vi "Get All Folder VI Data.vi"(8 "error in":errorcluster, 11 "Path":path) -> (0 "error out":errorcluster, 2 "Tree Map out":refnum<class "Tree Map.lvclass">, 3 "VI Data Map":T1)   [LabVIEW 2023, in "VI Properties Editor.lvlib"]
doc: "Gets all VI data from a folder located at <B>Path</B>."
uses:
  VI Properties Editor.lvlib
  Tree Map/Tree Map/Tree Map.lvclass
  <vilib>/picture/picture.llb/imagedata.ctl
  CTLs/VI Properties.ctl
  CTLs/Control Properties.ctl
  CTLs/VI Data Map.ctl
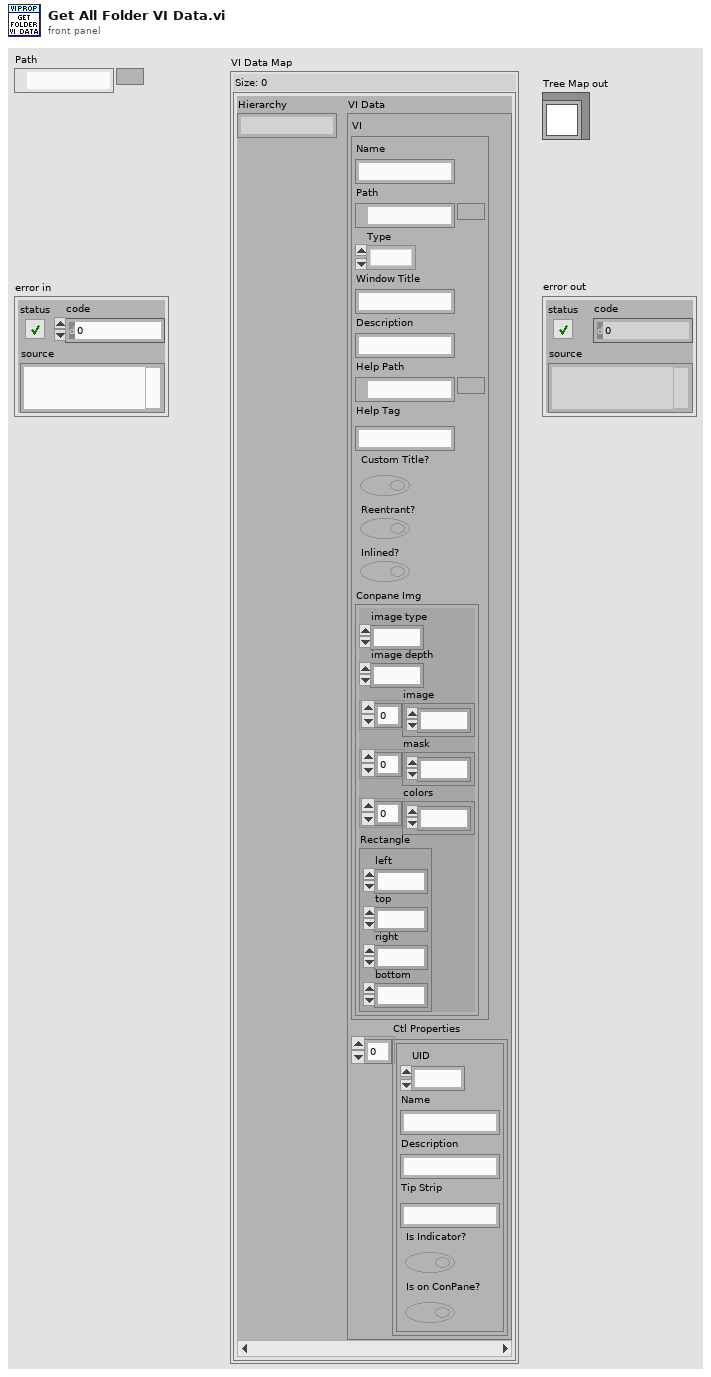
[diagram p1: front panel]
types:
  T1 = typedef "VI Properties Editor.lvlib/VI Data Map.ctl" = map{string, cluster{"VI":T2, "Ctl Properties":T4[]}}
  T2 = typedef "VI Properties Editor.lvlib/VI Properties.ctl" = cluster{"Name":string, "Path":path, "Type":enum32{"invalid VI type", "Standard VI", "Control VI", "Global VI", "Polymorphic VI", "Configuration VI", "SubSystem", "Facade VI", "Method VI", "Statechart Diagram VI"}, "Window Title":string, "Description":string, "Help Path":path, "Help Tag":string, "Custom Title?":bool, "Reentrant?":bool, "Inlined?":bool, "Conpane Img":T3}
  T3 = typedef "imagedata.ctl" = cluster{"image type":i32, "image depth":i32, "image":u8[], "mask":u8[], "colors":u32[], "Rectangle":cluster{"left":i16, "top":i16, "right":i16, "bottom":i16}}
  T4 = typedef "VI Properties Editor.lvlib/Control Properties.ctl" = cluster{"UID":i32, "Name":string, "Description":string, "Tip Strip":string, "Is Indicator?":bool, "Is on ConPane?":bool}
  T5 = typedef "VI Properties Editor.lvlib/VI Data.ctl" = cluster{"VI":T2, "Ctl Properties":T4[]}
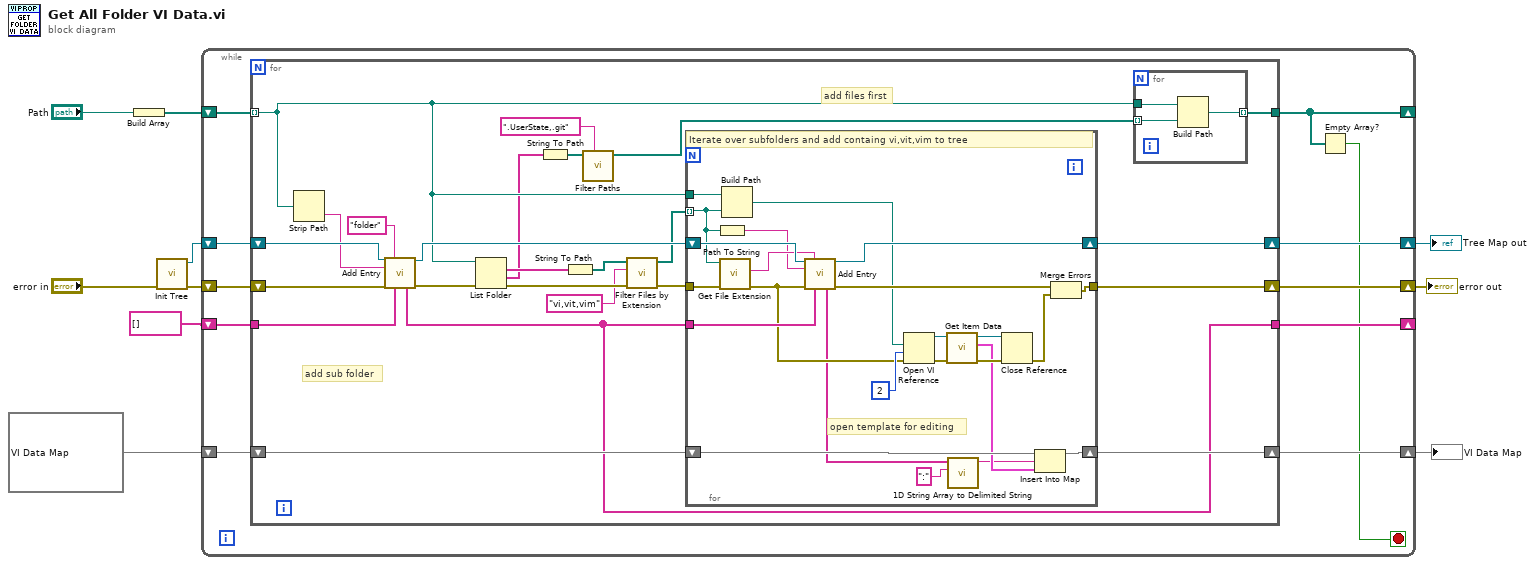
[diagram p0: block diagram]
diagram:
  n1 = Build Array("Path") -> (w3:path[])
  n2 = call "Init Tree.vi"("error in"="error in") -> ("error out"=w7:errorcluster, "Tree Map out"=w6:refnum<class "Tree Map.lvclass">)  [unwired: 9 in]
  n3 = while {
    shift-right: [w21] -> w10
    shift-left: w7 -> [w18]
    shift-right: [w20] -> w9
    shift-left: T1 {} ("VI Data Map") -> [w19]
    shift-right: [w15] -> w5
    shift-left: w6 -> [w16]
    shift-right: [w12] -> _
    shift-left: w3 -> [w14]
    shift-right: [w13] -> _
    shift-left: string[] [] ("Hierarchy") -> [w17]
    stop <- w11 stop-if-true
    n4 = for {
      tunnel: w17 -> [w29]
      tunnel: w14 -> [w28] mode=indexing
      shift-right: [w34] -> w21
      shift-left: w18 -> [w43]
      shift-right: [w39] -> w15
      shift-left: w16 -> [w41]
      shift-right: [w45] -> w20
      shift-left: w19 -> [w44]
      tunnel: [w26] -> w13
      tunnel: [w35] -> w12
      # "add files first"
      # "add sub folder"
      n5 = Strip Path(path=w28) -> (name=w27:string)  [unwired: 1 out]
      n6 = call "Add Entry.vi"("Tree Map in"=w41, "Symbol"="folder", "Name"=w27, "error in"=w43, "Parent (None)"=w29) -> ("Tree Map out"=w40:refnum<class "Tree Map.lvclass">, "Hierarchy"=w26:string[], "error out"=w42:errorcluster)  [unwired: 8 in]
      n7 = List Folder(path=w28, error in=w42) -> (filenames=w37:string[], folder names=w25:string[], error out=w32:errorcluster)  [unwired: 2 in, 1 out]
      n8 = String To Path(string=w25) -> (path=w23:path[])
      n9 = String To Path(string=w37) -> (path=w36:path[])
      n10 = call "Filter Paths.vi"("Argument"=".UserState,.git", "Paths"=w23) -> ("Filtered Path"=w24:path[])  [unwired: 9 in]
      n11 = call "Filter Files by Extension.vi"("error in (no error)"=w32, "Extensions"="vi,vit,vim", "Files"=w36) -> ("error out"=w31:errorcluster, "Files out"=w33:path[])  [unwired: 7 in]
      n12 = for {
        tunnel: w31 -> [w55]
        tunnel: [w53] -> w34
        shift-right: [w65] -> w45
        shift-left: w44 -> [w64]
        tunnel: w33 -> [w47] mode=indexing
        shift-right: [w61] -> w39
        shift-left: w40 -> [w62]
        tunnel: w26 -> [w56]
        tunnel: w28 -> [w49]
        # "open template for editing"
        # "Iterate over subfolders and add containg vi,vit,vim to tree"
        n13 = Path To String(path=w47) -> (string=w48:string)
        n14 = call <vilib>:"Get File Extension.vi"("error in (no error)"=w55, "file"=w47) -> ("error out"=w54:errorcluster, "lowercase file extension"=w60:string)  [unwired: 5 in, 3 out]
        n15 = Build Path(base path=w49, name or relative path=w47) -> (appended path=w46:path)
        n16 = call "Add Entry.vi"("Tree Map in"=w62, "Symbol"=w60, "Name"=w48, "error in"=w54, "Parent (None)"=w56) -> ("Tree Map out"=w61:refnum<class "Tree Map.lvclass">, "Hierarchy"=w50:string[], "error out"=w57:errorcluster)  [unwired: 8 in]
        n17 = Open VI Reference(vi path=w46, options=2, error in (no error)=w54) -> (vi reference=w67:refnum<vi>, error out=w68:errorcluster)  [unwired: 3 in]
        n18 = call "Get Item Data.vi"("error in (no error)"=w68, "VI Ref"=w67) -> ("error out"=w66:errorcluster, "VI Data"=w63:T5, "VI Ref out"=w51:refnum<vi>)  [unwired: 7 in]
        n19 = call <vilib>:"1D String Array to Delimited String.vi"("delimiter"=":", "string array"=w50) -> ("delimited string"=w58:string)  [unwired: 9 in]
        n20 = Close Reference(reference=w51, error in (no error)=w66) -> (error out=w52:errorcluster)
        n21 = Insert Into Map(map in=w64, key=w58, value=w63) -> (map out=w65:T1)  [unwired: 2 out]
        n22 = Merge Errors(w57, w52) -> (w53:errorcluster)
      }
      n23 = for {
        tunnel: w28 -> [w71]
        tunnel: w24 -> [w72] mode=indexing
        tunnel: [w70] -> w35 mode=indexing
        n24 = Build Path(base path=w71, name or relative path=w72) -> (appended path=w70:path)
      }
    }
    n25 = Empty Array?(array=w12) -> (empty?=w11:bool)
  }
  "VI Data Map" <- w9
  "error out" <- w10
  "Tree Map out" <- w5
